vi "CC_PI_testing.vi"() -> ()   [LabVIEW 2019]
uses:
  <vilib>/rvi/Emulation/niFpgaGetClockAttributes.vi
  <vilib>/rvi/Emulation/niFpgaSctlEmulationGetInTimedLoop.vi
  <vilib>/rvi/Emulation/niFpgaEmulationReportErrorSimple.vi
  <vilib>/rvi/eio/common/nirviEmuTemplateMethod_errors.vi
  <vilib>/rvi/Emulation/niFpgaCriticalErrorInLSC.vi
  <vilib>/eio/EIONode/EIONode.xnode
  <vilib>/rvi/Arithmetic/AddSubMult/XNode/nirviSatArithmetic.xnode
panel:
  in  "Position Reset joint side":bool
  in  "Velocity Interval (uSec)  joint side":u32=1000
  out "Position (Counts) joint side":i32(graph)
  out "Acceleration (Counts/Interval)  joint side":i32
  out "Velocity (Counts/Interval)  joint side":i32
  out "Loop time (position)  joint side":u32
  in  "weighting term encoder joint":sgl
  out "filtered joint position radians":sgl(graph)
  in  "Position Reset motor side":bool
  in  "Velocity Interval (uSec)  motor side":u32=1000
  out "Position (Counts) motor side":i32(graph)
  out "Acceleration (Counts/Interval)  motor side":i32
  out "Velocity (Counts/Interval)  motor side":i32
  out "Loop time (position)  motor side":u32
  in  "weighting term encoder motor":sgl
  out "filtered motor position radians":sgl(graph)
  out "error %":sgl(knob) scale=-100.0..100.0
  out "Loop rate":u16
  out "control_ip":sgl(graph)
  out "motor direction":bool
  in  "Ki":sgl
  in  "Kp":sgl
  in  "reference":sgl
  out "raw current":sgl
  in  "zero Value M2":sgl=2.4882812 format="%#_13g"
  out "Filtered Current(M2)":sgl(graph)
  in  "weighting term(M2)":sgl
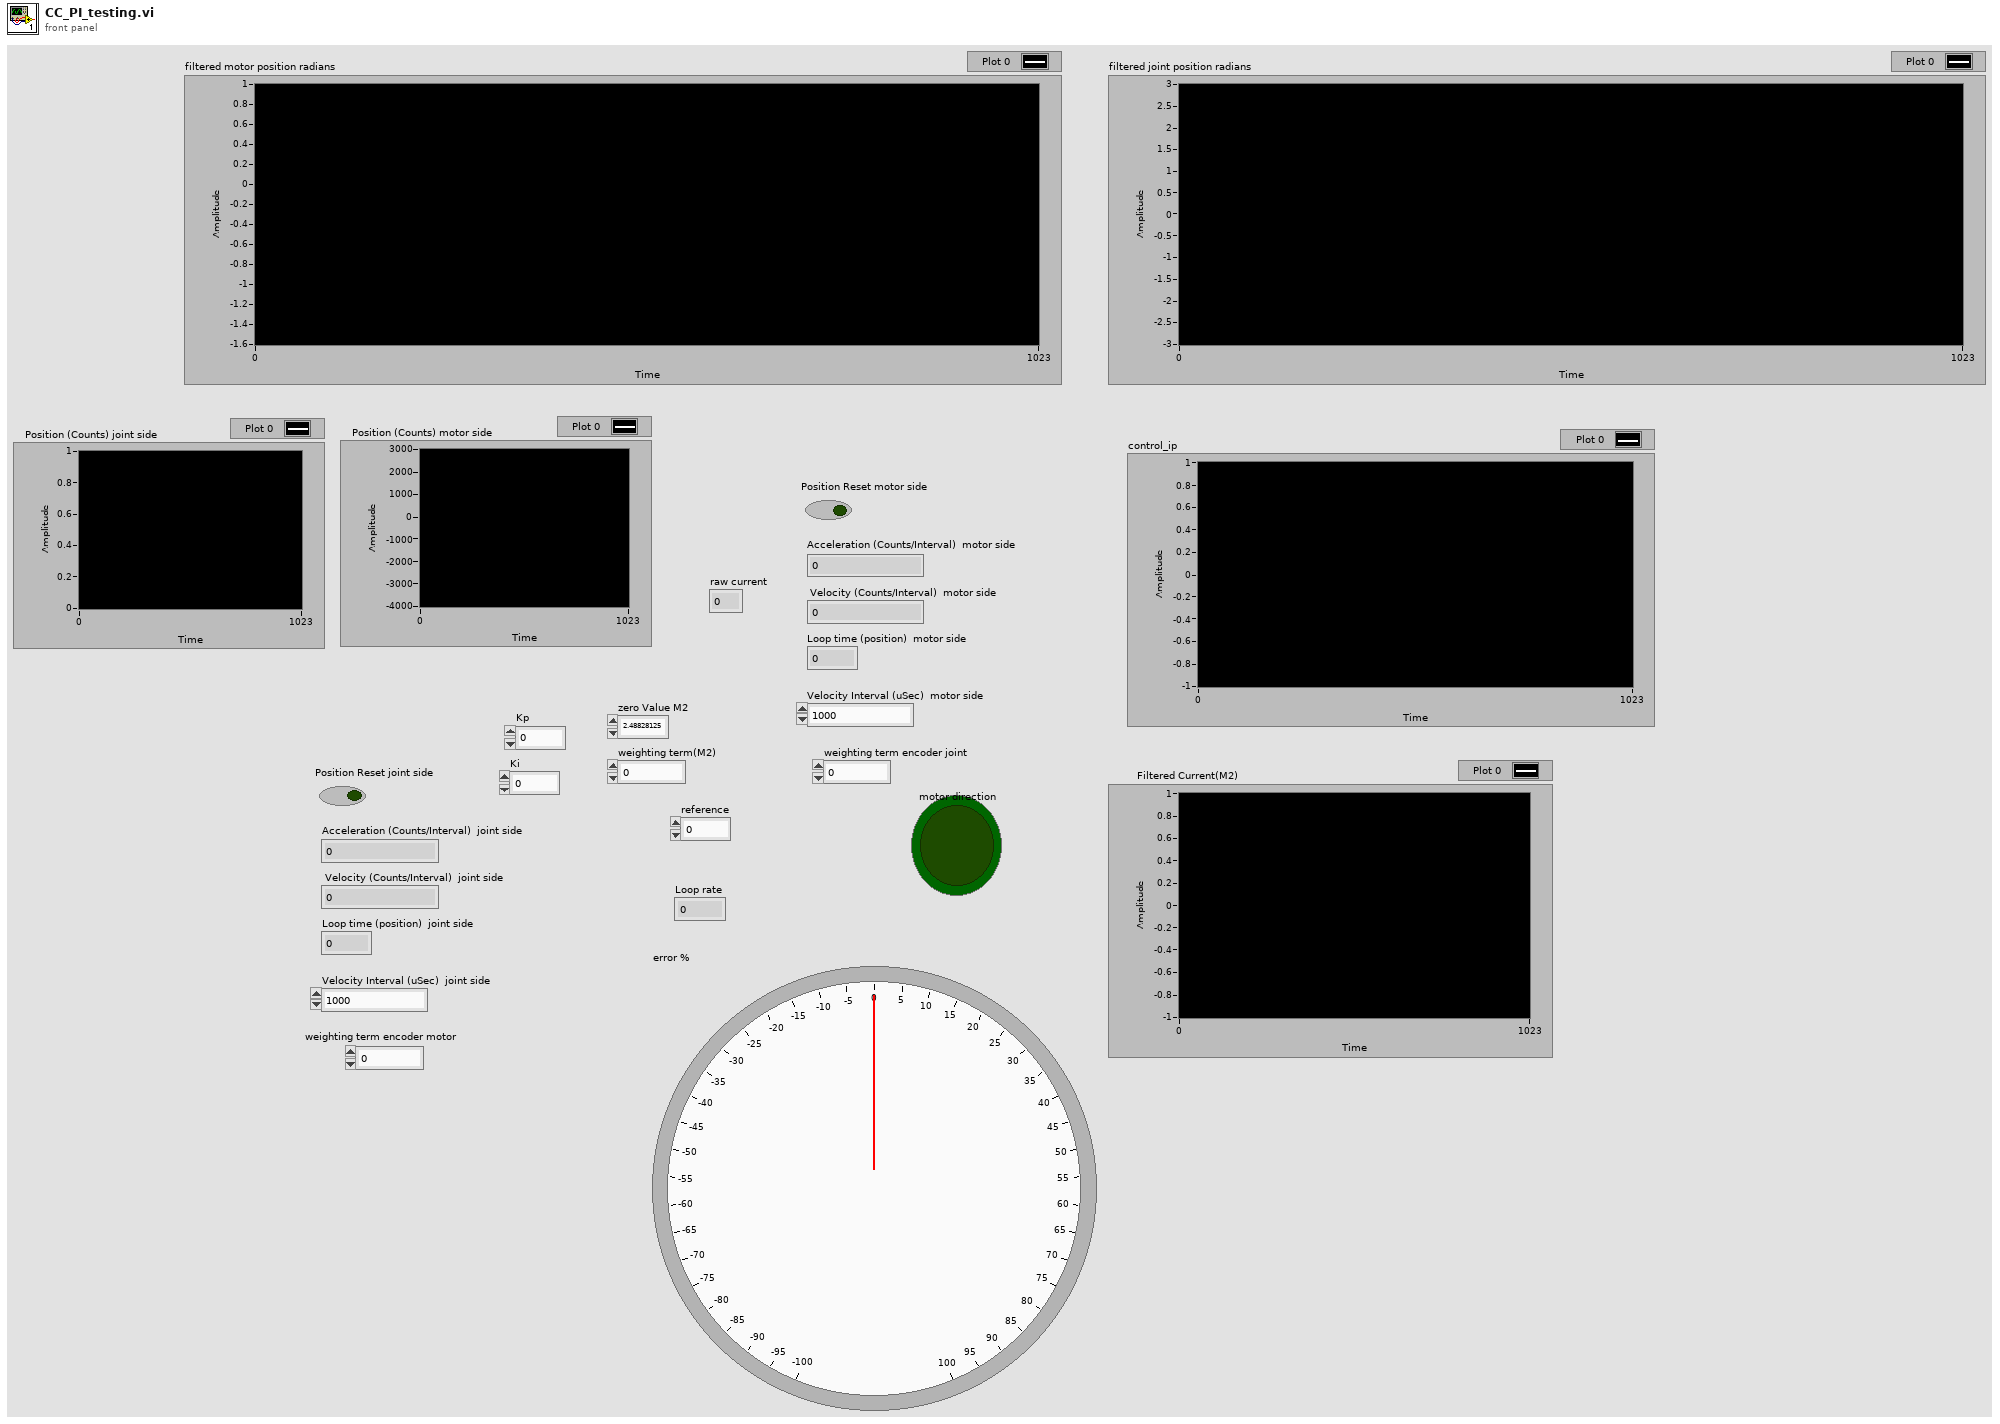
[diagram p1: front panel]
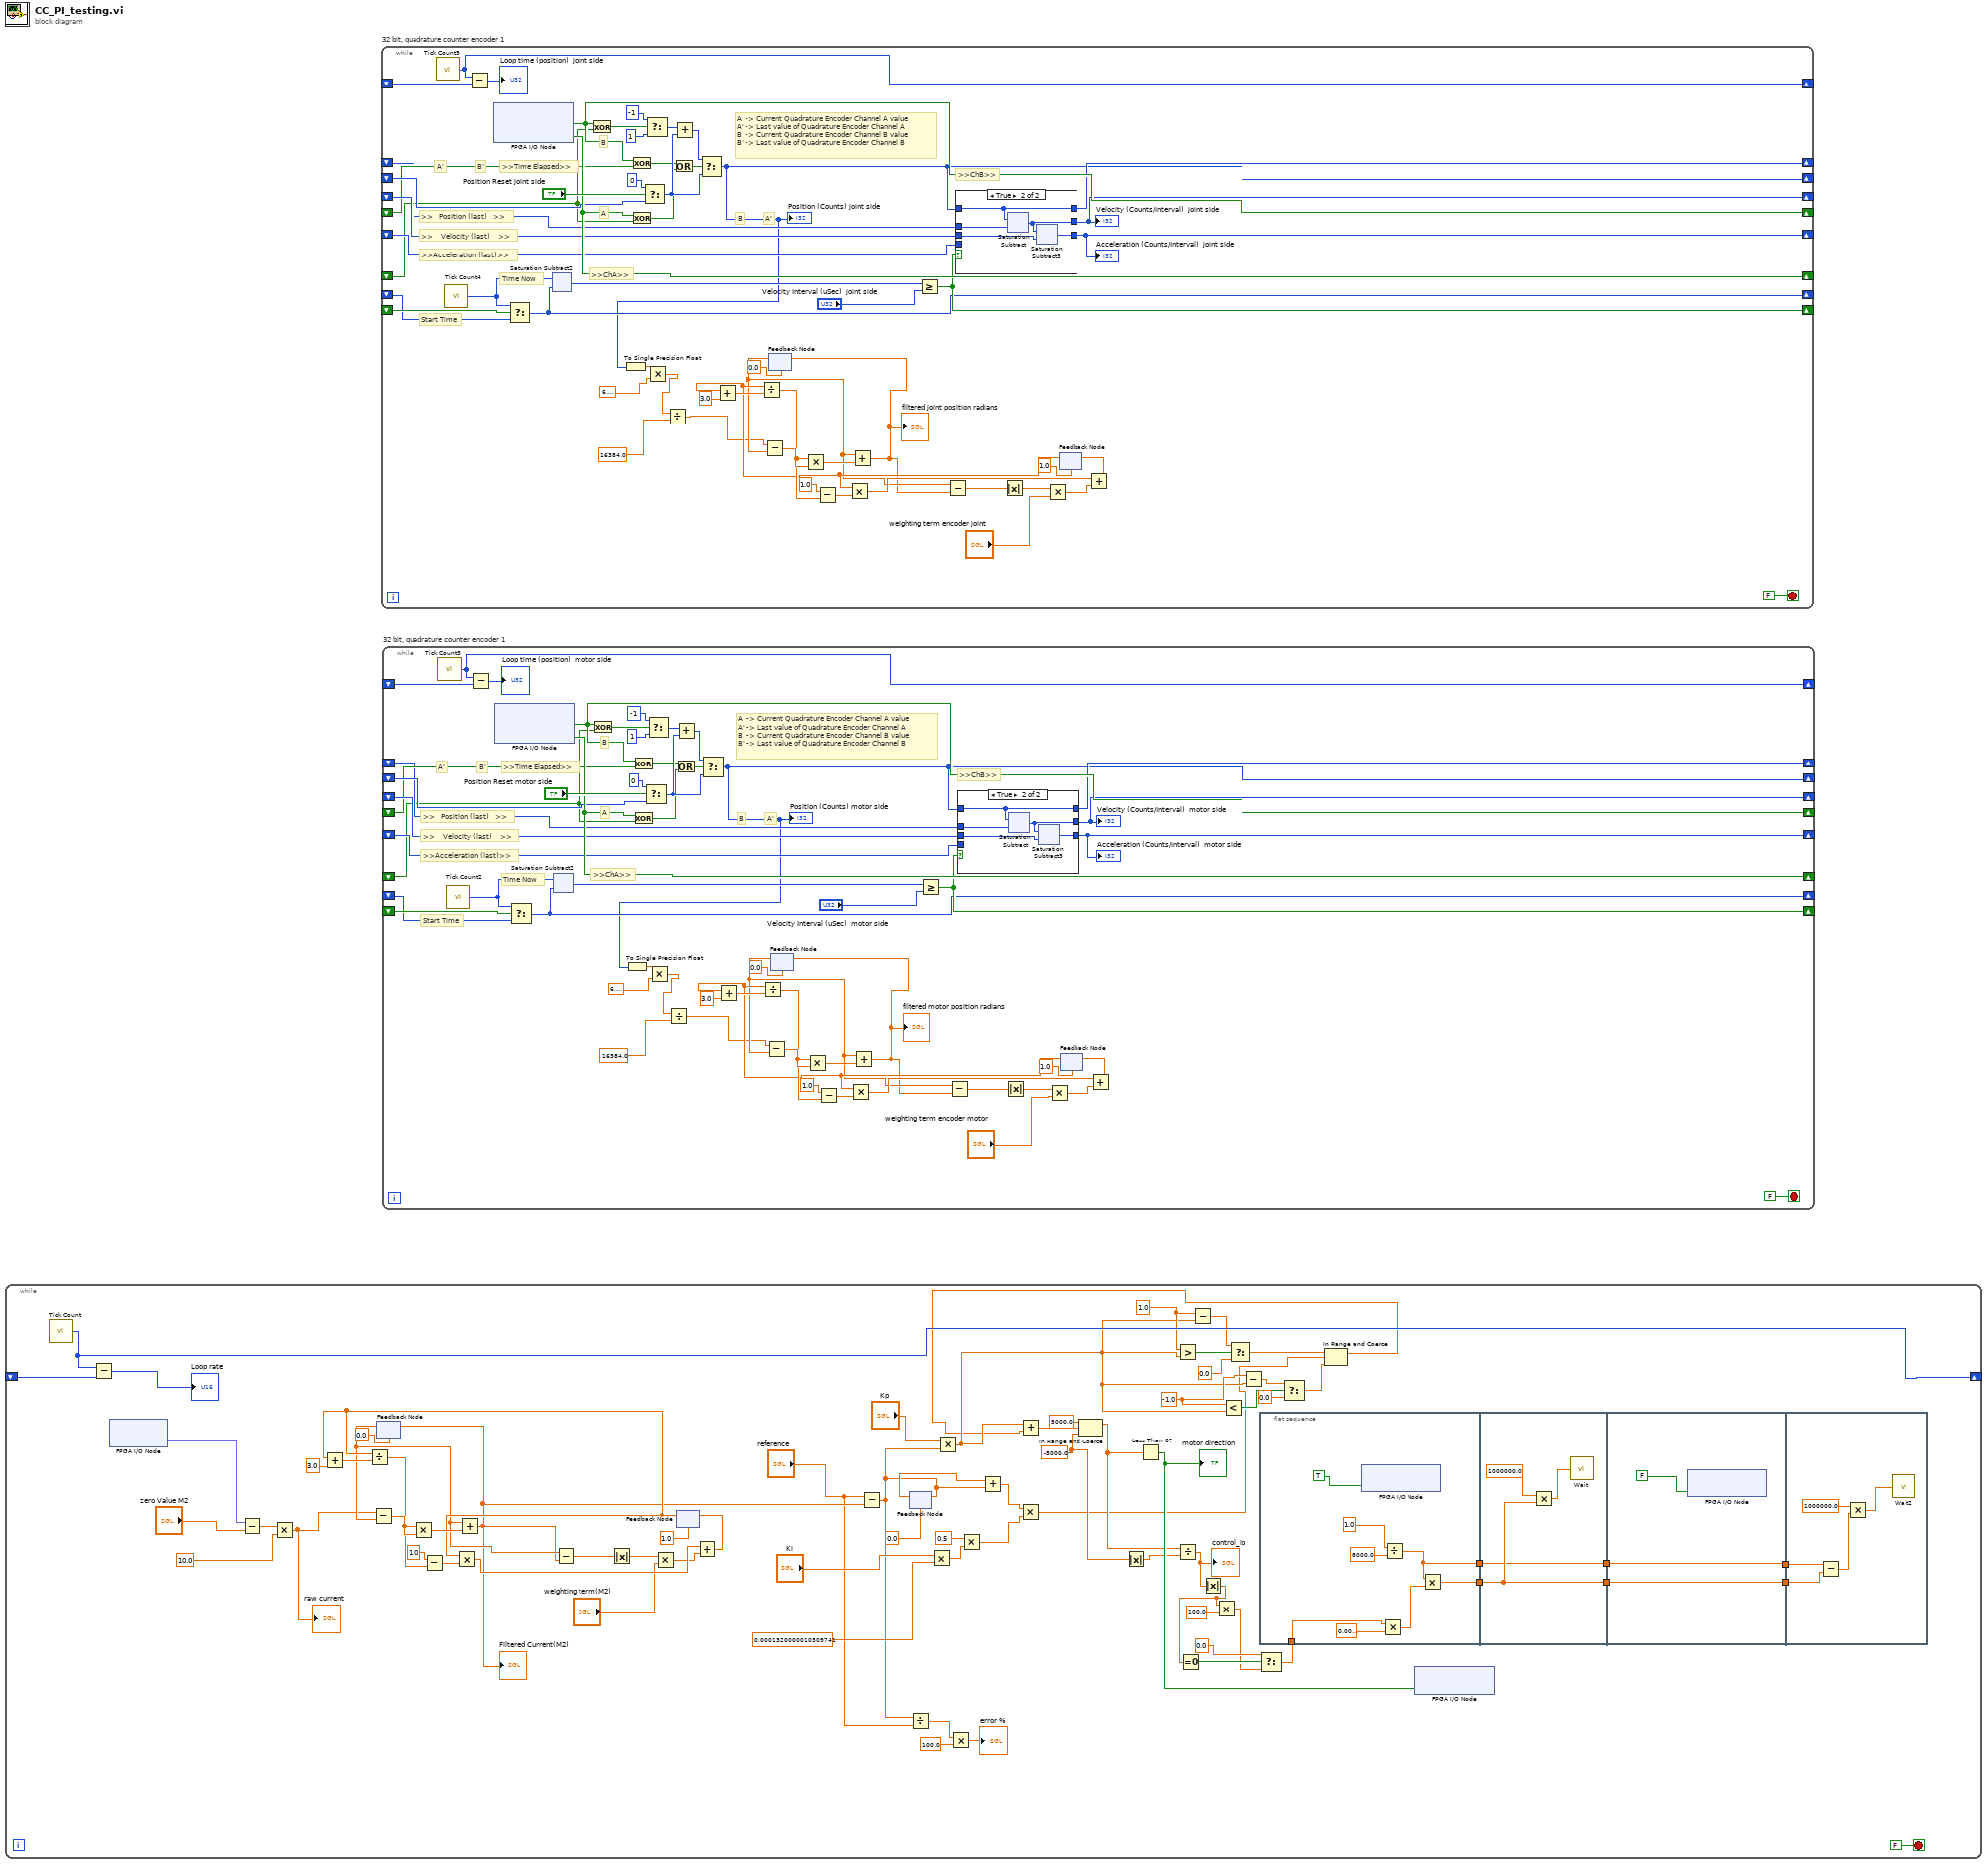
[diagram p0: block diagram]
diagram:
  n1 = while {
    shift-right: [w29] -> _
    shift-left: _ -> [w30]
    stop <- FALSE stop-if-true
    w2 = sgl -5000.0 ("lower limit")
    w8 = sgl -1.0 ("x")
    w11 = sgl 1.0 ("x")
    n2 = call "Tick Count"() -> ("Tick Count(uSec)"=w29:u16)
    n3 = Subtract(x=w29, y=w30) -> (x-y=→"Loop rate":u16)
    n4 = xnode "FPGA I/O Node"() -> ("AI0"=w52:fxp<+/-,24,5>)  [unwired: 1 in, 1 out]
    n5 = Subtract(x=w52, y="zero Value M2") -> (x-y=w53:sgl)
    n6 = Multiply(x=w53, y=sgl 10.0) -> (x*y=w55:sgl)
    "raw current" <- w55
    n7 = feedback #1(sgl 0.0) -> (w63:sgl)
    n8 = Subtract(x=w55, y=w63) -> (x-y=w71:sgl)
    n9 = feedback #2(sgl 1.0) -> (w64:sgl)
    n10 = Add(x=w64, y=sgl 3.0) -> (x+y=w73:sgl)
    n11 = Divide(x=w64, y=w73) -> (x/y=w70:sgl)
    n12 = Multiply(x=w70, y=w71) -> (x*y=w72:sgl)
    n13 = Subtract(x=sgl 1.0, y=w70) -> (x-y=w69:sgl)
    n14 = Multiply(x=w64, y=w69) -> (x*y=w68:sgl)
    n15 = Add(x=w63, y=w72) -> (x+y=w51:sgl)
    "Filtered Current(M2)" <- w51
    n16 = feedback-in #1(w51) -> ()
    n17 = Subtract(x=w63, y=w51) -> (x-y=w67:sgl)
    n18 = Absolute Value(x=w67) -> (abs(x)=w66:sgl)
    n19 = Multiply(x=w66, y="weighting term(M2)") -> (x*y=w65:sgl)
    n20 = Add(x=w68, y=w65) -> (x+y=w57:sgl)
    n21 = feedback-in #2(w57) -> ()
    n22 = Subtract(x="reference", y=w51) -> (x-y=w27:sgl)
    n23 = feedback-in #3(w27) -> ()
    n24 = feedback #3(sgl 0.0) -> (w46:sgl)
    n25 = Divide(x=w27, y="reference") -> (x/y=w19:sgl)
    n26 = Multiply(x="Ki", y=sgl 0.000132) -> (x*y=w48:sgl)
    n27 = Multiply(x="Kp", y=w27) -> (x*y=w7:sgl)
    n28 = Multiply(x=w19, y=sgl 100.0) -> (x*y=→"error %":sgl)
    n29 = Multiply(x=sgl 0.5, y=w48) -> (x*y=w44:sgl)
    n30 = Add(x=w46, y=w27) -> (x+y=w45:sgl)
    n31 = Multiply(x=w45, y=w44) -> (x*y=w1:sgl)
    n32 = Absolute Value(x=w2) -> (abs(x)=w31:sgl)
    n33 = Greater?(x=w11, y=w7) -> (0:w16:bool)
    n34 = Subtract(x=w11, y=w7) -> (x-y=w15:sgl)
    n35 = Less?(x=w8, y=w7) -> (x < y?=w10:bool)
    n36 = Select(t=w15, s=w16, f=sgl 0.0) -> (s? t:f=w13:sgl)
    n37 = Subtract(x=w8, y=w7) -> (x-y=w9:sgl)
    n38 = flat-sequence {
      tunnel: [w78] -> w40
      tunnel: [w76] -> w39
      tunnel: w21 -> [w74]
      tunnel: w40 -> [w83]
      tunnel: [w83] -> w38
      tunnel: w39 -> [w82]
      tunnel: [w82] -> w37
      tunnel: w38 -> [w88]
      tunnel: [w88] -> w36
      tunnel: w37 -> [w87]
      tunnel: [w87] -> w35
      tunnel: w36 -> [w93]
      tunnel: w35 -> [w89]
      frame #0 {
        n39 = xnode "FPGA I/O Node"("RMC/DIO50"=TRUE) -> ()  [unwired: 1 in, 1 out]
        n40 = Multiply(x=w74, y=sgl 0.01) -> (x*y=w79:sgl)
        n41 = Divide(x=sgl 1.0, y=sgl 8000.0) -> (x/y=w76:sgl)
        n42 = Multiply(x=w76, y=w79) -> (x*y=w78:sgl)
      }
      frame #1 {
        n43 = Multiply(x=sgl 1000000.0, y=w83) -> (x*y=w85:sgl)
        n44 = call "Wait"("Count(uSec)"=w85) -> ()  [unwired: 1 out]
      }
      frame #2 {
        n45 = xnode "FPGA I/O Node"("RMC/DIO50"=FALSE) -> ()  [unwired: 1 in, 1 out]
      }
      frame #3 {
        n46 = Subtract(x=w89, y=w93) -> (x-y=w92:sgl)
        n47 = Multiply(x=sgl 1000000.0, y=w92) -> (x*y=w91:sgl)
        n48 = call "Wait2"("Count(uSec)"=w91) -> ()  [unwired: 1 out]
      }
    }
    n49 = Select(t=w9, s=w10, f=sgl 0.0) -> (s? t:f=w5:sgl)
    n50 = In Range and Coerce(upper limit=w13, x=w1, lower limit=w5) -> (coerced(x)=w4:sgl)  [unwired: 1 out]
    n51 = Add(x=w7, y=w4) -> (x+y=w41:sgl)
    n52 = In Range and Coerce(upper limit=sgl 5000.0, x=w41, lower limit=w2) -> (coerced(x)=w12:sgl)  [unwired: 1 out]
    n53 = Less Than 0?(x=w12) -> (x < 0?=w34:bool)
    "motor direction" <- w34
    n54 = Divide(x=w12, y=w31) -> (x/y=w33:sgl)
    "control_ip" <- w33
    n55 = Absolute Value(x=w33) -> (abs(x)=w24:sgl)
    n56 = Equal To 0?(x=w24) -> (x = 0?=w25:bool)
    n57 = Multiply(x=w24, y=sgl 100.0) -> (x*y=w22:sgl)
    n58 = Select(t=sgl 0.0, s=w25, f=w22) -> (s? t:f=w21:sgl)
    n59 = xnode "FPGA I/O Node"("RMC/DIO54"=w34) -> ()  [unwired: 1 in, 1 out]
  }
  n60 = while "32 bit, quadrature counter encoder 1" {
    shift-right: [w140] -> _
    shift-left: _ -> [w127]
    shift-right: [w98] -> _
    shift-left: _ -> [w137]
    shift-right: [w139] -> _
    shift-left: _ -> [w118]
    shift-right: [w133] -> _
    shift-left: _ -> [w136]
    shift-right: [w129] -> _
    shift-left: _ -> [w134]
    shift-right: [w124] -> _
    shift-left: _ -> [w123]
    shift-right: [w125] -> _
    shift-left: _ -> [w131]
    shift-right: [w126] -> _
    shift-left: _ -> [w128]
    shift-right: [w120] -> _
    shift-left: _ -> [w122]
    stop <- FALSE stop-if-true
    # "A  -> Current Quadrature Encoder Channel A value\nA' -> Last value of Quadrature Encoder Channel A\nB  -> Current Quadrature Encoder Channel B value\nB' -> Last value of Quadrature Encoder Channel B"
    # ">>Acceleration (last)>>"
    # "Start Time"
    # "A'"
    # "B"
    # "A'"
    # "A"
    # "B'"
    # "B"
    # ">>ChB>>"
    # ">>ChA>>"
    # ">>    Velocity (last)    >>"
    # ">>   Position (last)   >>"
    # "Time Now"
    # ">>Time Elapsed>>"
    n61 = call "Tick Count5"() -> ("Tick Count(uSec)"=w120:u32)
    n62 = call "Tick Count4"() -> ("Tick Count(uSec)"=w130:u32)
    n63 = Subtract(x=w120, y=w122) -> (x-y=→"Loop time (position)  joint side":u32)
    n64 = xnode "FPGA I/O Node"() -> ("RMC/DIO44"=w140:bool, "RMC/DIO42"=w139:bool)  [unwired: 2 in, 2 out]
    n65 = Select(t=w130, s=w136, f=w134) -> (s? t:f=w129:u32)
    n66 = xnode ("Saturation Subtract2")("x"=w130, "y"=w129) -> ("x-y"=w132:u32)
    n67 = Exclusive Or(1:w118, 2:w140) -> (0:w141:bool)
    n68 = Exclusive Or(1:w127, 2:w140) -> (0:w142:bool)
    n69 = Exclusive Or(1:w118, 2:w139) -> (0:w143:bool)
    n70 = Select(t=0 ("32 bit"), s="Position Reset joint side", f=w137) -> (s? t:f=w148:i32)
    n71 = Select(t=-1 ("32 bit"), s=w141, f=1 ("32 bit")) -> (s? t:f=w146:i32)
    n72 = Add(x=w146, y=w148) -> (x+y=w150:i32)
    n73 = Or(x=w142, y=w143) -> (x .or. y?=w138:bool)
    n74 = Select(t=w150, s=w138, f=w148) -> (s? t:f=w98:i32)
    "Position (Counts) joint side" <- w98
    n75 = To Single Precision Float(number=w98) -> (single precision float=w99:sgl)
    n76 = Multiply(x=w99, y=sgl 6.2831855) -> (x*y=w97:sgl)
    n77 = Divide(x=w97, y=sgl 16384.0) -> (x/y=w95:sgl)
    n78 = feedback #4(sgl 0.0) -> (w107:sgl)
    n79 = Subtract(x=w95, y=w107) -> (x-y=w115:sgl)
    n80 = Greater Or Equal?(x=w132, y="Velocity Interval (uSec)  joint side") -> (x >= y?=w133:bool)
    n81 = case shown="True" w133 {
      tunnel: w98 -> [_ w164]
      tunnel: w123 -> [w161 w168]
      tunnel: [w163 w167] -> w125
      tunnel: w131 -> [w163 w166]
      tunnel: [w162 w165] -> w126
      tunnel: w128 -> [w162 _]
      tunnel: [w161 w164] -> w124
      frame False {
      }
      frame True {
        n82 = xnode ("Saturation Subtract")("x"=w164, "y"=w168) -> ("x-y"=w167:i32)
        n83 = xnode ("Saturation Subtract3")("x"=w167, "y"=w166) -> ("x-y"=w165:i32)
      }
    }
    "Acceleration (Counts/Interval)  joint side" <- w126
    "Velocity (Counts/Interval)  joint side" <- w125
    n84 = feedback #5(sgl 1.0) -> (w108:sgl)
    n85 = Add(x=w108, y=sgl 3.0) -> (x+y=w117:sgl)
    n86 = Divide(x=w108, y=w117) -> (x/y=w114:sgl)
    n87 = Multiply(x=w114, y=w115) -> (x*y=w116:sgl)
    n88 = Subtract(x=sgl 1.0, y=w114) -> (x-y=w113:sgl)
    n89 = Multiply(x=w108, y=w113) -> (x*y=w112:sgl)
    n90 = Add(x=w107, y=w116) -> (x+y=w100:sgl)
    "filtered joint position radians" <- w100
    n91 = feedback-in #4(w100) -> ()
    n92 = Subtract(x=w107, y=w100) -> (x-y=w111:sgl)
    n93 = Absolute Value(x=w111) -> (abs(x)=w110:sgl)
    n94 = Multiply(x=w110, y="weighting term encoder joint") -> (x*y=w109:sgl)
    n95 = Add(x=w112, y=w109) -> (x+y=w102:sgl)
    n96 = feedback-in #5(w102) -> ()
  }
  n97 = while "32 bit, quadrature counter encoder 1" {
    shift-right: [w251] -> _
    shift-left: _ -> [w238]
    shift-right: [w209] -> _
    shift-left: _ -> [w248]
    shift-right: [w250] -> _
    shift-left: _ -> [w229]
    shift-right: [w244] -> _
    shift-left: _ -> [w247]
    shift-right: [w240] -> _
    shift-left: _ -> [w245]
    shift-right: [w235] -> _
    shift-left: _ -> [w234]
    shift-right: [w236] -> _
    shift-left: _ -> [w242]
    shift-right: [w237] -> _
    shift-left: _ -> [w239]
    shift-right: [w231] -> _
    shift-left: _ -> [w233]
    stop <- FALSE stop-if-true
    # "A  -> Current Quadrature Encoder Channel A value\nA' -> Last value of Quadrature Encoder Channel A\nB  -> Current Quadrature Encoder Channel B value\nB' -> Last value of Quadrature Encoder Channel B"
    # ">>Acceleration (last)>>"
    # "Start Time"
    # "A'"
    # "B"
    # "A'"
    # "A"
    # "B'"
    # "B"
    # ">>ChB>>"
    # ">>ChA>>"
    # ">>    Velocity (last)    >>"
    # ">>   Position (last)   >>"
    # "Time Now"
    # ">>Time Elapsed>>"
    n98 = call "Tick Count3"() -> ("Tick Count(uSec)"=w231:u32)
    n99 = call "Tick Count2"() -> ("Tick Count(uSec)"=w241:u32)
    n100 = Subtract(x=w231, y=w233) -> (x-y=→"Loop time (position)  motor side":u32)
    n101 = xnode "FPGA I/O Node"() -> ("RMC/DIO40"=w251:bool, "RMC/DIO38"=w250:bool)  [unwired: 2 in, 2 out]
    n102 = Select(t=w241, s=w247, f=w245) -> (s? t:f=w240:u32)
    n103 = xnode ("Saturation Subtract2")("x"=w241, "y"=w240) -> ("x-y"=w243:u32)
    n104 = Exclusive Or(1:w229, 2:w251) -> (0:w252:bool)
    n105 = Exclusive Or(1:w238, 2:w251) -> (0:w253:bool)
    n106 = Exclusive Or(1:w229, 2:w250) -> (0:w254:bool)
    n107 = Select(t=0 ("32 bit"), s="Position Reset motor side", f=w248) -> (s? t:f=w259:i32)
    n108 = Select(t=-1 ("32 bit"), s=w252, f=1 ("32 bit")) -> (s? t:f=w257:i32)
    n109 = Add(x=w257, y=w259) -> (x+y=w261:i32)
    n110 = Or(x=w253, y=w254) -> (x .or. y?=w249:bool)
    n111 = Select(t=w261, s=w249, f=w259) -> (s? t:f=w209:i32)
    "Position (Counts) motor side" <- w209
    n112 = To Single Precision Float(number=w209) -> (single precision float=w210:sgl)
    n113 = Multiply(x=w210, y=sgl 6.2831855) -> (x*y=w208:sgl)
    n114 = Divide(x=w208, y=sgl 16384.0) -> (x/y=w206:sgl)
    n115 = feedback #6(sgl 0.0) -> (w218:sgl)
    n116 = Subtract(x=w206, y=w218) -> (x-y=w226:sgl)
    n117 = Greater Or Equal?(x=w243, y="Velocity Interval (uSec)  motor side") -> (x >= y?=w244:bool)
    n118 = case shown="True" w244 {
      tunnel: w209 -> [_ w275]
      tunnel: w234 -> [w272 w279]
      tunnel: [w274 w278] -> w236
      tunnel: w242 -> [w274 w277]
      tunnel: [w273 w276] -> w237
      tunnel: w239 -> [w273 _]
      tunnel: [w272 w275] -> w235
      frame False {
      }
      frame True {
        n119 = xnode ("Saturation Subtract")("x"=w275, "y"=w279) -> ("x-y"=w278:i32)
        n120 = xnode ("Saturation Subtract3")("x"=w278, "y"=w277) -> ("x-y"=w276:i32)
      }
    }
    "Acceleration (Counts/Interval)  motor side" <- w237
    "Velocity (Counts/Interval)  motor side" <- w236
    n121 = feedback #7(sgl 1.0) -> (w219:sgl)
    n122 = Add(x=w219, y=sgl 3.0) -> (x+y=w228:sgl)
    n123 = Divide(x=w219, y=w228) -> (x/y=w225:sgl)
    n124 = Multiply(x=w225, y=w226) -> (x*y=w227:sgl)
    n125 = Subtract(x=sgl 1.0, y=w225) -> (x-y=w224:sgl)
    n126 = Multiply(x=w219, y=w224) -> (x*y=w223:sgl)
    n127 = Add(x=w218, y=w227) -> (x+y=w211:sgl)
    "filtered motor position radians" <- w211
    n128 = feedback-in #6(w211) -> ()
    n129 = Subtract(x=w218, y=w211) -> (x-y=w222:sgl)
    n130 = Absolute Value(x=w222) -> (abs(x)=w221:sgl)
    n131 = Multiply(x=w221, y="weighting term encoder motor") -> (x*y=w220:sgl)
    n132 = Add(x=w223, y=w220) -> (x+y=w213:sgl)
    n133 = feedback-in #7(w213) -> ()
  }
